vi "filter.volume.data.vi"(4 "colors":T1, 5 "Show All":bool, 6 "Threshold":dbl=0.8, 7 "Volume Type":T2, 8 "storyArcs":string[](array[string])=["cyclops", "phoenix", "beast", "iceman", "angel", "jean grey", "nightcrawler", "storm", "wolverine", "colossus", "banshee", "kitty pryde"], 9 "characters":string[](array[string])=["cyclops", "phoenix", "beast", "iceman", "angel", "jean grey", "nightcrawler", "storm", "wolverine", "colossus", "banshee", "kitty pryde"], 10 "team":string[](array[string])=["x-men", "x-factor", "x-force", "new mutants"], 11 "volume_map":T3[](array[typedef])) -> (0 "end date":timestamp, 1 "start date":timestamp, 2 "found":i32, 3 "sorted volume objects":cluster{"Array":T5[]}[](array[cluster]))   [LabVIEW 2024]
uses:
  volume.object--cluster.ctl
  volume.map--cluster.ctl
  definitions/volume.type--enum.ctl
  <vilib>/Utility/error.llb/Trim Whitespace One-Sided.vi
panel:
  out "size(s)":i32
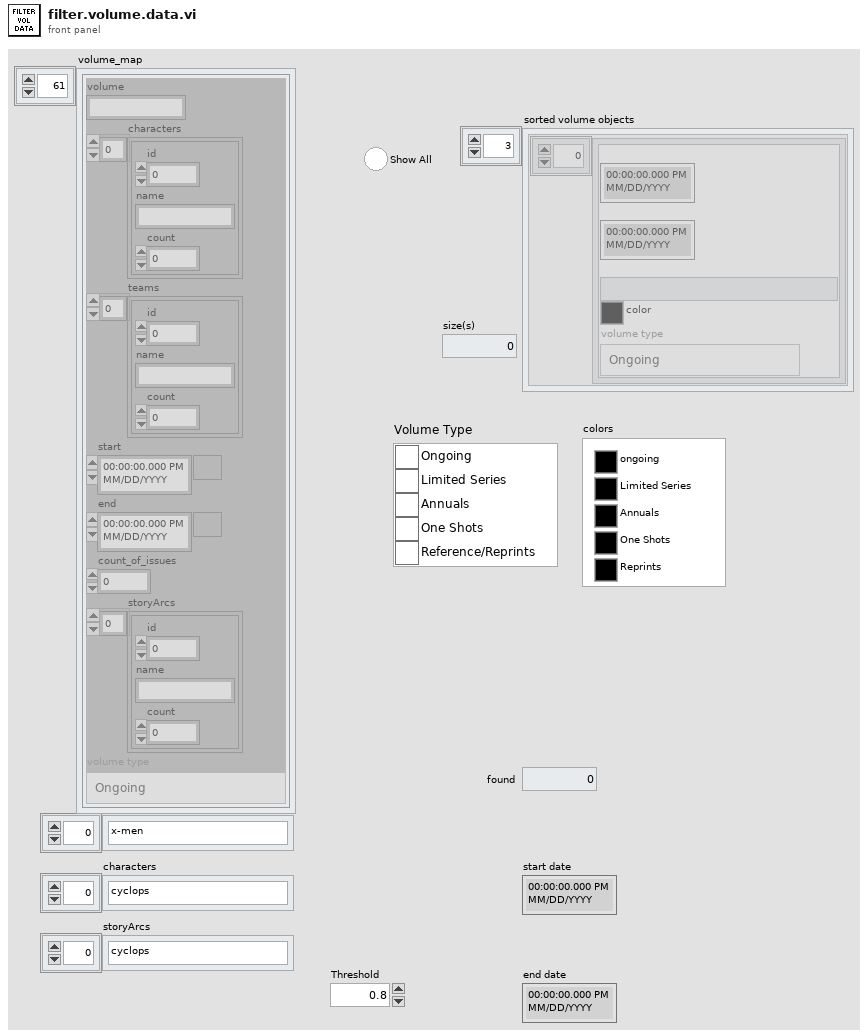
[diagram p1: front panel]
types:
  T1 = cluster{"ongoing":u32, "Limited Series":u32, "Annuals":u32, "One Shots":u32, "Reprints":u32}
  T2 = cluster{"Ongoing":bool, "Limited Series":bool, "Annuals":bool, "One Shots":bool, "Reference/Reprints":bool}
  T3 = typedef "volume.map--cluster.ctl" = cluster{"volume":string, "characters":cluster{"id":i32, "name":string, "count":i32}[], "teams":cluster{"id":i32, "name":string, "count":i32}[], "start":timestamp, "end":timestamp, "count_of_issues":i32, "storyArcs":cluster{"id":i32, "name":string, "count":i32}[], "volume type":T4}
  T4 = typedef "volume.type--enum.ctl" = enum16{"Ongoing", "Limited Series", "Annual", "One Shot", "Reprint/Document"}
  T5 = typedef "volume.object--cluster.ctl" = cluster{"start date":timestamp, "end date":timestamp, "sortable_name":string, "color":u32, "volume type":T4}
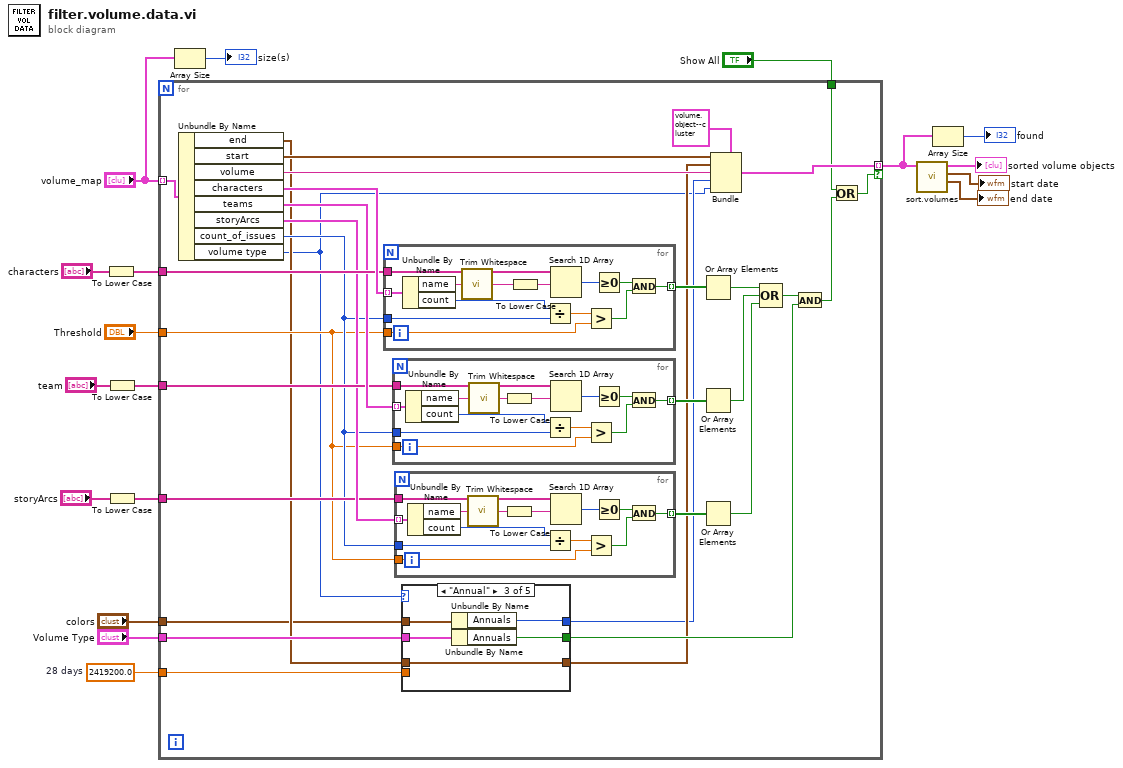
[diagram p0: block diagram]
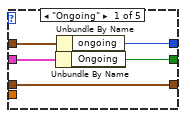
[diagram p2: hidden frame]
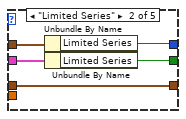
[diagram p3: hidden frame]
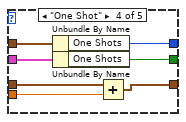
[diagram p4: hidden frame]
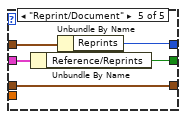
[diagram p5: hidden frame]
diagram:
  w10 = 2419200.0  # 28 days
  n1 = To Lower Case(string="characters") -> (all lower case string=w7:string[])
  n2 = To Lower Case(string="team") -> (all lower case string=w6:string[])
  n3 = To Lower Case(string="storyArcs") -> (all lower case string=w4:string[])
  n4 = for {
    tunnel: "volume_map" -> [w48] mode=indexing
    tunnel: "Threshold" -> [w34]
    tunnel: w6 -> [w42]
    tunnel: [w49] -> w14 mode=indexing if=w20
    tunnel: w7 -> [w44]
    tunnel: w10 -> [w26]
    tunnel: w4 -> [w36]
    tunnel: "Volume Type" -> [w31]
    tunnel: "colors" -> [w25]
    tunnel: "Show All" -> [w22]
    n5 = Unbundle By Name(w48) -> ("end"=w28:timestamp, "start"=w46:timestamp, "volume"=w45:string, "characters"=w47:cluster{"id":i32, "name":string, "count":i32}[], "teams"=w43:cluster{"id":i32, "name":string, "count":i32}[], "storyArcs"=w37:cluster{"id":i32, "name":string, "count":i32}[], "count_of_issues"=w35:i32, "volume type"=w19:T4)
    n6 = for {
      tunnel: w47 -> [w88] mode=indexing
      tunnel: w44 -> [w86]
      tunnel: w35 -> [w83]
      tunnel: w34 -> [w81]
      tunnel: [w78] -> w41 mode=indexing
      n7 = Unbundle By Name(w88) -> ("name"=w87:string, "count"=w84:i32)
      n8 = call <vilib>:"Trim Whitespace.vi"("string"=w87) -> ("trimmed string"=w76:string)  [unwired: 1 in]
      n9 = To Lower Case(string=w76) -> (all lower case string=w77:string)
      n10 = Divide(x=w84, y=w83) -> (x/y=w82:dbl)
      n11 = Search 1D Array(1D array=w86, element=w77) -> (index of element=w85:i32)  [unwired: 1 in]
      n12 = Greater?(x=w82, y=w81) -> (0:w79:bool)
      n13 = Greater Or Equal To 0?(x=w85) -> (x >= 0?=w80:bool)
      n14 = And(x=w80, y=w79) -> (x .and. y?=w78:bool)
    }
    n15 = for {
      tunnel: w43 -> [w75] mode=indexing
      tunnel: w42 -> [w73]
      tunnel: w35 -> [w70]
      tunnel: w34 -> [w68]
      tunnel: [w65] -> w40 mode=indexing
      n16 = Unbundle By Name(w75) -> ("name"=w74:string, "count"=w71:i32)
      n17 = call <vilib>:"Trim Whitespace.vi"("string"=w74) -> ("trimmed string"=w63:string)  [unwired: 1 in]
      n18 = To Lower Case(string=w63) -> (all lower case string=w64:string)
      n19 = Divide(x=w71, y=w70) -> (x/y=w69:dbl)
      n20 = Search 1D Array(1D array=w73, element=w64) -> (index of element=w72:i32)  [unwired: 1 in]
      n21 = Greater?(x=w69, y=w68) -> (0:w66:bool)
      n22 = Greater Or Equal To 0?(x=w72) -> (x >= 0?=w67:bool)
      n23 = And(x=w67, y=w66) -> (x .and. y?=w65:bool)
    }
    n24 = for {
      tunnel: w37 -> [w62] mode=indexing
      tunnel: w36 -> [w60]
      tunnel: w35 -> [w57]
      tunnel: w34 -> [w55]
      tunnel: [w52] -> w33 mode=indexing
      n25 = Unbundle By Name(w62) -> ("name"=w61:string, "count"=w58:i32)
      n26 = call <vilib>:"Trim Whitespace.vi"("string"=w61) -> ("trimmed string"=w50:string)  [unwired: 1 in]
      n27 = To Lower Case(string=w50) -> (all lower case string=w51:string)
      n28 = Divide(x=w58, y=w57) -> (x/y=w56:dbl)
      n29 = Search 1D Array(1D array=w60, element=w51) -> (index of element=w59:i32)  [unwired: 1 in]
      n30 = Greater?(x=w56, y=w55) -> (0:w53:bool)
      n31 = Greater Or Equal To 0?(x=w59) -> (x >= 0?=w54:bool)
      n32 = And(x=w54, y=w53) -> (x .and. y?=w52:bool)
    }
    n33 = case shown="\"Annual\"" w19 {
      tunnel: w31 -> [w93 w98 w103 w110 w115]
      tunnel: [w92 w97 w102 w109 w114] -> w29
      tunnel: w28 -> [w91 w96 w101 w107 w113]
      tunnel: [w91 w96 w101 w106 w113] -> w27
      tunnel: w26 -> [_ _ _ w108 _]
      tunnel: w25 -> [w90 w95 w100 w105 w112]
      tunnel: [w89 w94 w99 w104 w111] -> w24
      frame "Ongoing" {
        n34 = Unbundle By Name(w93) -> ("Ongoing"=w92:bool)
        n35 = Unbundle By Name(w90) -> ("ongoing"=w89:u32)
      }
      frame "Limited Series" {
        n36 = Unbundle By Name(w95) -> ("Limited Series"=w94:u32)
        n37 = Unbundle By Name(w98) -> ("Limited Series"=w97:bool)
      }
      frame "Annual" {
        n38 = Unbundle By Name(w100) -> ("Annuals"=w99:u32)
        n39 = Unbundle By Name(w103) -> ("Annuals"=w102:bool)
      }
      frame "One Shot" {
        n40 = Unbundle By Name(w105) -> ("One Shots"=w104:u32)
        n41 = Unbundle By Name(w110) -> ("One Shots"=w109:bool)
        n42 = Add(x=w107, y=w108) -> (x+y=w106:timestamp)
      }
      frame "Reprint/Document" {
        n43 = Unbundle By Name(w115) -> ("Reference/Reprints"=w114:bool)
        n44 = Unbundle By Name(w112) -> ("Reprints"=w111:u32)
      }
    }
    n45 = Or Array Elements(Boolean array=w41) -> (logical OR=w39:bool)
    n46 = Or Array Elements(Boolean array=w40) -> (logical OR=w38:bool)
    n47 = Or Array Elements(Boolean array=w33) -> (logical OR=w32:bool)
    n48 = Bundle(cluster=T5 {"start date"=timestamp(0 s since 1904-01-01), "end date"=timestamp(0 s since 1904-01-01), "sortable_name"="", "color"=0, "volume type"=enum."Ongoing"} ("Cluster"), "start date"=w46, "end date"=w27, "sortable_name"=w45, "color"=w24, "volume type"=w19) -> (w49:T5)
    n49 = Compound Arithmetic op=OR(w39, w38, w32) -> (w30:bool)
    n50 = And(x=w30, y=w29) -> (x .and. y?=w21:bool)
    n51 = Or(x=w22, y=w21) -> (x .or. y?=w20:bool)
  }
  n52 = Array Size(array="volume_map") -> (size(s)=→"size(s)":i32)
  n53 = call "sort.volumes.vi"("volumes"=w14) -> ("end date"=→"end date":timestamp, "start date"=→"start date":timestamp, "Array"=→"sorted volume objects":cluster{"Array":T5[]}[])  [unwired: 8 in]
  n54 = Array Size(array=w14) -> (size(s)=→"found":i32)
